vi "signal_cut.vi"(8 "error in":errorcluster, 9 "hammerIndex":i32, 10 "data":dbl[][](array[numeric]), 11 "config":T2 {"updateTime" format="%#_g ms"; "lowPass" format="%#_g Hz"; "highPass" format="%#_g Hz"; "cutoff" format="%#_g dB"; "preTrigger" format="%#_g ms"; "thr" format="%#_g N"; "duration" format="%#_g s"; "rate" min=1652.0 max=51200.0 format="%#_g Hz"}) -> (0 "error out":errorcluster, 3 "data_out":T1 {"config"."updateTime" format="%#_g ms"; "config"."lowPass" format="%#_g Hz"; "config"."highPass" format="%#_g Hz"; "config"."cutoff" format="%#_g dB"; "config"."preTrigger" format="%#_g ms"; "config"."thr" format="%#_g N"; "config"."duration" format="%#_g s"; "config"."rate" min=1652.0 max=51200.0 format="%#_g Hz"})   [LabVIEW 2017]
uses:
  MainFGV/Settings/Advanced/AdvancedConfig.ctl
  results_data.ctl
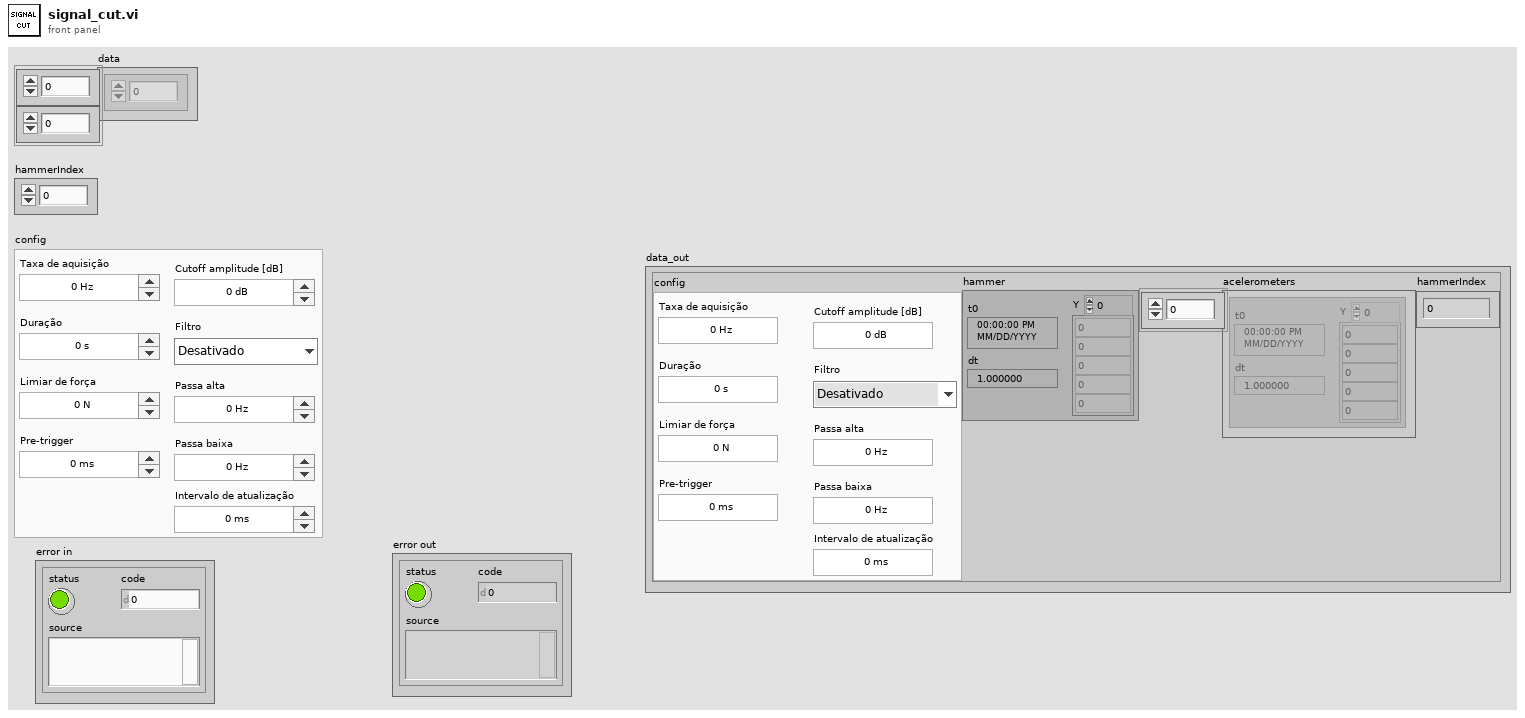
[diagram p1: front panel]
types:
  T1 = typedef "results_data.ctl" = cluster{"config":T2, "hammer":waveform(dbl), "acelerometers":waveform(dbl)[], "hammerIndex":i32}
  T2 = typedef "AdvancedConfig.ctl" = cluster{"rate":dbl, "duration":dbl, "thr":dbl, "preTrigger":dbl, "cutoff":dbl, "Filtro":enum16{"Desativado", "Passa banda", "Passa alta", "Passa baixa"}, "highPass":dbl, "lowPass":dbl, "updateTime":dbl}
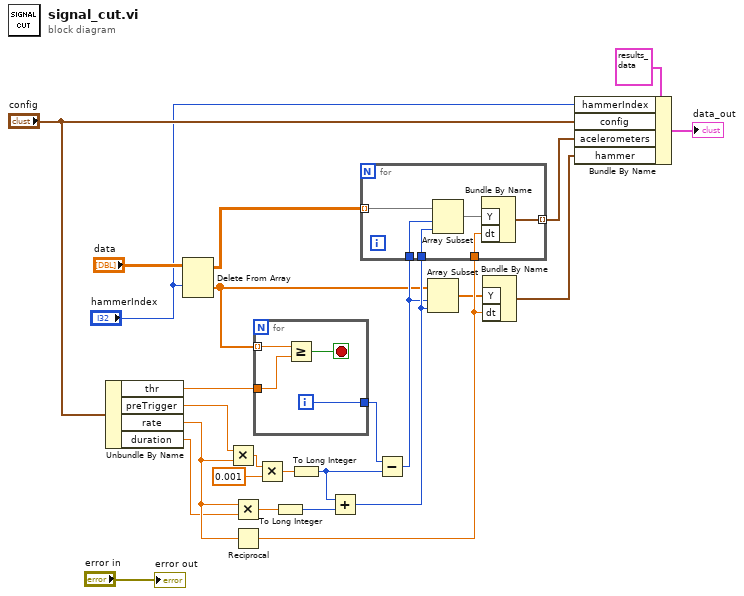
[diagram p0: block diagram]
diagram:
  n1 = Unbundle By Name("config") -> ("thr"=w9:dbl, "preTrigger"=w10:dbl, "rate"=w20:dbl, "duration"=w15:dbl)
  n2 = Delete From Array(array="data", index (row)="hammerIndex") -> (deleted portion=w21:dbl[], array with subset deleted=w22:dbl[][])  [unwired: 2 in]
  n3 = Multiply(x=w10, y=w20) -> (x*y=w11:dbl)
  n4 = Multiply(x=w20, y=w15) -> (x*y=w16:dbl)
  n5 = Reciprocal(x=w20) -> (1/x=w25:dbl)
  n6 = for {
    tunnel: w21 -> [w29] mode=indexing
    tunnel: w9 -> [w28]
    tunnel: [w26] -> w14
    i -> [w26]
    stop <- w27 stop-if-true
    n7 = Greater Or Equal?(x=w29, y=w28) -> (x >= y?=w27:bool)
  }
  n8 = Multiply(x=w11, y=0.001) -> (x*y=w13:dbl)
  n9 = To Long Integer(number=w16) -> (32bit integer=w17:i32)
  n10 = To Long Integer(number=w13) -> (32bit integer=w18:i32)
  n11 = Add(x=w18, y=w17) -> (x+y=w24:i32)
  n12 = Subtract(x=w14, y=w18) -> (x-y=w23:i32)
  n13 = for {
    tunnel: w22 -> [w35] mode=indexing
    tunnel: w23 -> [w34]
    tunnel: w24 -> [w33]
    tunnel: w25 -> [w31]
    tunnel: [w30] -> w5 mode=indexing
    n14 = Array Subset(array=w35, index=w34, length=w33) -> (w32:dbl[])
    n15 = Bundle By Name("Y"=w32, "dt"=w31) -> (w30:waveform(dbl))  [unwired: 1 in]
  }
  n16 = Array Subset(array=w21, index=w23, length=w24) -> (w19:dbl[])
  n17 = Bundle By Name("Y"=w19, "dt"=w25) -> (w4:waveform(dbl))  [unwired: 1 in]
  n18 = Bundle By Name(cluster=T1 {"config"={"rate"=0.0, "duration"=0.0, "thr"=0.0, "preTrigger"=0.0, "cutoff"=0.0, "Filtro"=enum."Desativado", "highPass"=0.0, "lowPass"=0.0, "updateTime"=0.0}, "hammer"={"t0"=timestamp(0 s since 1904-01-01), "dt"=1.0, "Y"=[]}, "acelerometers"=[], "hammerIndex"=0} ("results_data"), "hammerIndex"="hammerIndex", "config"="config", "acelerometers"=w5, "hammer"=w4) -> (→"data_out":T1)
  "error out" <- "error in"
